vi "test RT Config - Single RT Sweep.vi"(8 "error in (no error)":errorcluster, 11 "RT Config in":refnum<class "RT Config.lvclass">) -> (0 "error out":errorcluster, 3 "RT Config out":refnum<class "RT Config.lvclass">)   [LabVIEW 2016, in "RT Config.lvclass"]
uses:
  RT Config.lvclass
  1553 Board/1553 Board.lvclass
  1553 Component/1553 Component.lvclass
  Remote Terminal/Remote Terminal.lvclass
  Remote Terminal/TypeDefs/RT Configuration.ctl
  1553 SubComponent/TypeDefs/Scaling Information.ctl
  1553 SubComponent/1553 SubComponent.lvclass
  1553 SubComponent/TypeDefs/Parameter Table Data.ctl
  Remote Terminal/TypeDefs/Command Type.ctl
  Remote Terminal/TypeDefs/Command Configuration.ctl
  D:/SVN/Products/BCI-1553/Software/Development/2016/RealTime/1553 SubComponent/1553 SubComponent.lvclass
  PPLs/FPGA Interface.lvlibp/FPGA Interface/FPGA Interface.lvclass
  Utilities/FPGA Interface/FPGA Interface.lvclass
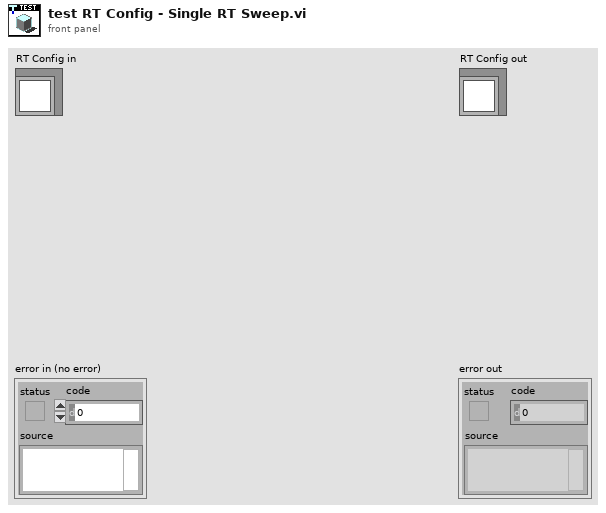
[diagram p1: front panel]
types:
  T1 = typedef "BCI-1553 API.lvlib/Remote Terminal.lvclass/RT Configuration.ctl" = cluster{"RT-RT TimeOut (us)":u8, "Inhibit Bus A":bool, "Inhibit Bus B":bool, "Broadcast CMD Invalid":bool, "UnDef MCs Invalid":bool, "Notice 2 Data Storage":bool, "SMCP":bool, "Temp RX Buffer":bool, "Alt BIT Enable":bool, "Auto Bus Shutdown":bool, "MC 17 Sync":u8, "MC 16 SR Reset":bool, "MC 8 Reset":bool}
  T2 = typedef "BCI-1553 API.lvlib/Remote Terminal.lvclass/Command Type.ctl" = enum16{"Transmit", "Receive", "Mode Code Tx", "Mode Code Rx"}
  T3 = typedef "BCI-1553 API.lvlib/Remote Terminal.lvclass/Command Configuration.ctl" = cluster{"Command Type":T2, "Mode Code ID (1-32)":u16, "SubAddress (1-30)":u16, "Word Count (1-32)":u16, "Illegal Command":bool, "Broadcast":bool, "Data":u16[], "Data Fields":T4[]}
  T4 = typedef "BCI-1553 API.lvlib/1553 SubComponent.lvclass/Parameter Table Data.ctl" = cluster{"Parameter Name":string, "Base Word":u16, "Address":u16, "Value":u64, "Mask":u16[], "Scaling Info":T5}
  T5 = typedef "BCI-1553 API.lvlib/1553 SubComponent.lvclass/Scaling Information.ctl" = cluster{"Bit Offset":i32, "Bit Count":i32, "LSB Resolution":dbl, "2's Complement":bool, "Big Endian":bool, "Sign Bit":bool}
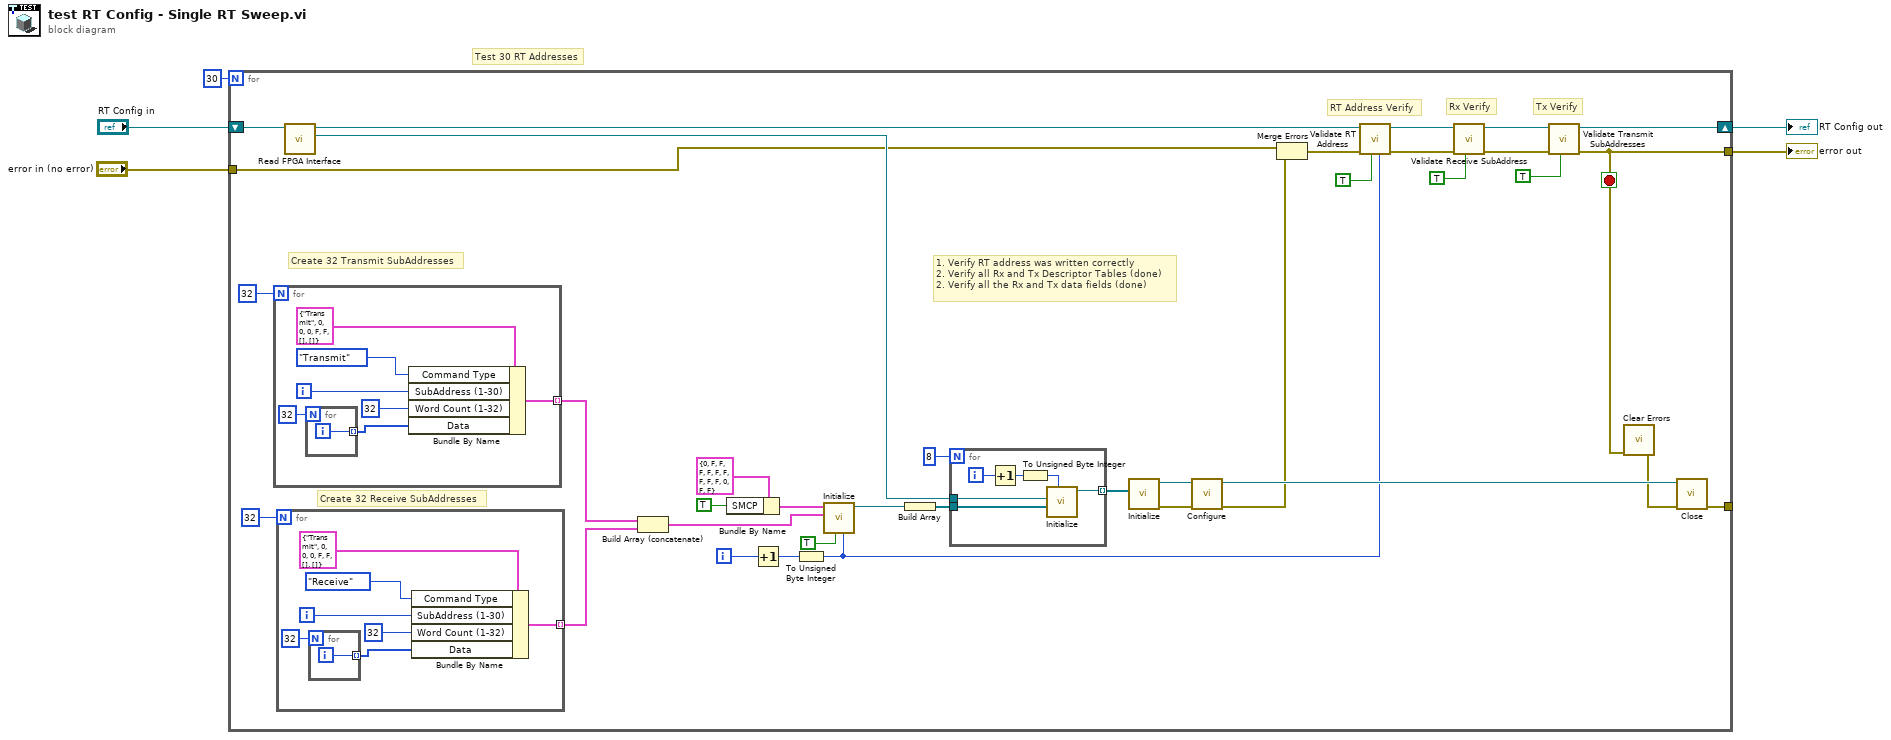
[diagram p0: block diagram]
diagram:
  # "Test 30 RT Addresses"
  n1 = for {
    N: 30 -> [_]
    shift-right: [w19] -> w1
    shift-left: "RT Config in" -> [w28]
    tunnel: [w26] -> _
    tunnel: "error in (no error)" -> [w16]
    tunnel: [w18] -> w2
    i -> [w30]
    stop <- w18 stop-if-true
    # "RT Address Verify"
    # "Rx Verify"
    # "Tx Verify"
    # "1. Verify RT address was written correctly\n2. Verify all Rx and Tx Descriptor Tables (done)\n2. Verify all the Rx and Tx data fields (done)"
    # "Create 32 Receive SubAddresses"
    # "Create 32 Transmit SubAddresses"
    n2 = for {
      N: 32 -> [_]
      tunnel: [w51] -> w21 mode=indexing
      i -> [w50]
      n3 = for {
        N: 32 -> [_]
        tunnel: [w57] -> w52 mode=indexing
        i -> [w57]
      }
      n4 = Bundle By Name(cluster=T3 {"Command Type"=enum."Transmit", "Mode Code ID (1-32)"=0, "SubAddress (1-30)"=0, "Word Count (1-32)"=0, "Illegal Command"=FALSE, "Broadcast"=FALSE, "Data"=[], "Data Fields"=[]} ("CMD Configuration"), "Command Type"=Command_Type."Transmit", "SubAddress (1-30)"=w50, "Word Count (1-32)"=u16 32, "Data"=w52) -> (w51:T3)
    }
    n5 = for {
      N: 32 -> [_]
      tunnel: [w43] -> w23 mode=indexing
      i -> [w42]
      n6 = for {
        N: 32 -> [_]
        tunnel: [w49] -> w44 mode=indexing
        i -> [w49]
      }
      n7 = Bundle By Name(cluster=T3 {"Command Type"=enum."Transmit", "Mode Code ID (1-32)"=0, "SubAddress (1-30)"=0, "Word Count (1-32)"=0, "Illegal Command"=FALSE, "Broadcast"=FALSE, "Data"=[], "Data Fields"=[]} ("CMD Configuration"), "Command Type"=Command_Type."Receive", "SubAddress (1-30)"=w42, "Word Count (1-32)"=u16 32, "Data"=w44) -> (w43:T3)
    }
    n8 = call-dynamic "Read FPGA Interface.vi"("1553 Test in"=w28) -> ("FPGA Interface"=w36:refnum<class "FPGA Interface.lvclass">, "1553 Test out"=w11:refnum<class "RT Config.lvclass">)  [unwired: 8 in, 1 out]
    n9 = Build Array (concatenate)(w21, w23) -> (w22:T3[])
    n10 = Bundle By Name(cluster=T1 {"RT-RT TimeOut (us)"=0, "Inhibit Bus A"=FALSE, "Inhibit Bus B"=FALSE, "Broadcast CMD Invalid"=FALSE, "UnDef MCs Invalid"=FALSE, "Notice 2 Data Storage"=FALSE, "SMCP"=FALSE, "Temp RX Buffer"=FALSE, "Alt BIT Enable"=FALSE, "Auto Bus Shutdown"=FALSE, "MC 17 Sync"=0, "MC 16 SR Reset"=FALSE, "MC 8 Reset"=FALSE} ("RT Configuration"), "SMCP"=TRUE) -> (w39:T1)
    n11 = Increment(x=w30) -> (x+1=w29:i32)
    n12 = To Unsigned Byte Integer(number=w29) -> (unsigned 8bit integer=w6:u8)
    n13 = call "Initialize.vi"("RT Address (0-30)"=w6, "RT 1?"=TRUE, "Commands"=w22, "RT Configuration"=w39) -> ("Remote Terminal out"=w38:refnum<class "Remote Terminal.lvclass">)  [unwired: 6 in, 1 out]
    n14 = Build Array(w38) -> (w37:refnum<class "Remote Terminal.lvclass">[])
    n15 = for {
      N: 8 -> [_]
      tunnel: [w61] -> w41 mode=indexing
      tunnel: w37 -> [w60]
      tunnel: w36 -> [w59]
      i -> [w63]
      n16 = Increment(x=w63) -> (x+1=w58:i32)
      n17 = To Unsigned Byte Integer(number=w58) -> (unsigned 8bit integer=w62:u8)
      n18 = call "Initialize.vi"("Component ID (1-8)"=w62, "SubComponents"=w60, "FPGA Interface"=w59) -> ("1553 Component out"=w61:refnum<class "1553 Component.lvclass">)  [unwired: 7 in, 1 out]
    }
    n19 = call "Initialize.vi"("Components"=w41) -> ("error out"=w31:errorcluster, "1553 Board out"=w32:refnum<class "1553 Board.lvclass">)  [unwired: 9 in]
    n20 = call-dynamic "Configure.vi"("error in (no error)"=w31, "1553 Board in"=w32) -> ("error out"=w15:errorcluster, "1553 Board out"=w27:refnum<class "1553 Board.lvclass">)  [unwired: 8 in]
    n21 = Merge Errors(w16, w15) -> (w9:errorcluster)
    n22 = call "Validate RT Address.vi"("RT Address (0-30)"=w6, "RT 1?"=TRUE, "error in (no error)"=w9, "RT Config in"=w11) -> ("error out"=w8:errorcluster, "RT Config out"=w10:refnum<class "RT Config.lvclass">)  [unwired: 6 in]
    n23 = call "Validate Receive SubAddress.vi"("RT 1?"=TRUE, "error in (no error)"=w8, "RT Config in"=w10) -> ("error out"=w13:errorcluster, "RT Config out"=w14:refnum<class "RT Config.lvclass">)  [unwired: 7 in]
    n24 = call "Validate Transmit SubAddresses.vi"("RT 1?"=TRUE, "error in (no error)"=w13, "RT Config in"=w14) -> ("error out"=w18:errorcluster, "RT Config out"=w19:refnum<class "RT Config.lvclass">)  [unwired: 7 in]
    n25 = call <vilib>:"Clear Errors.vi"("error in (no error)"=w18) -> ("error out"=w17:errorcluster)  [unwired: 5 in, 1 out]
    n26 = call-dynamic "Close.vi"("error in (no error)"=w17, "1553 Board in"=w27) -> ("error out"=w26:errorcluster)  [unwired: 9 in]
  }
  "error out" <- w2
  "RT Config out" <- w1
